vi "Hide_HMI.vi"(8 "error in (no error)":errorcluster caption="entrée d'erreur (pas d'erreur)", 11 "Class Popup (Default) en entrée":refnum<class "Class Popup (Main).lvclass">) -> (0 "error out":errorcluster caption="sortie d'erreur", 3 "Class Popup (Default) en sortie":refnum<class "Class Popup (Main).lvclass">)   [LabVIEW 2020, in "Library Instrument & Equipement.lvlib" / "Library Popup.lvlib" / "Class Popup (Main).lvclass"]
uses:
  Class Popup (Main).lvclass
  Class Popup (Main).lvclass/Class Popup (Main).ctl
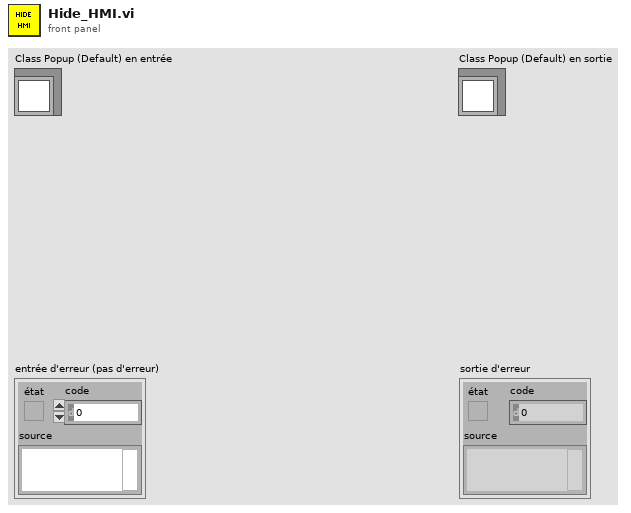
[diagram p1: front panel]
types:
  T1 = enum32{"Invalid", "Standard", "Closed", "Hidden", "Minimized", "Maximized"}
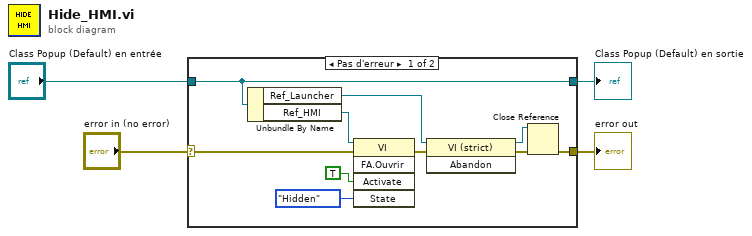
[diagram p0: block diagram]
diagram:
  n1 = case shown="Pas d'erreur" "error in (no error)" {
    selector: "error in (no error)" -> [w9 w16]
    tunnel: [w13 w16] -> w3
    tunnel: [w14 w15] -> w1
    tunnel: "Class Popup (Default) en entrée" -> [w14 w15]
    frame No Error {
      n2 = Unbundle By Name(w14) -> ("Ref_Launcher"=w12:refnum<vi>, "Ref_HMI"=w6:refnum<vi>)
      n3 = invoke class="VI" method="FA.Ouvrir"(reference=w6, error in=w9, "Activate"=TRUE ("Activer ?"), "State"=T1."Hidden" ("État")) -> (error out=w7:errorcluster)  [unwired: 1 in, 4 out]
      n4 = invoke class="VI (strict)" method="Abandon"(reference=w12, error in=w7) -> (reference out=w5:refnum<vi>, error out=w8:errorcluster)  [unwired: 1 in, 1 out]
      n5 = Close Reference(reference=w5, error in (no error)=w8) -> (error out=w13:errorcluster)
    }
    frame Error {
    }
  }
  "error out" <- w3
  "Class Popup (Default) en sortie" <- w1
